vi "Service Key.vi"(11 "Service In":refnum<class "Service.lvclass">) -> (2 "Service Key":string, 3 "Service":refnum<class "Service.lvclass">)   [LabVIEW 2020, in "HTTP Server.lvlib" / "Values.lvclass"]
uses:
  Values.lvclass
  Service/Service.lvclass
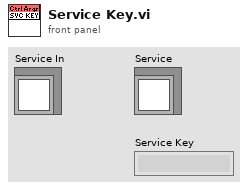
[diagram p1: front panel]
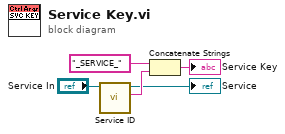
[diagram p0: block diagram]
diagram:
  n1 = call-dynamic "Service ID.vi"("Service in"="Service In") -> ("Service ID"=w4:string, "Service out"=→"Service":refnum<class "Service.lvclass">)  [unwired: 8 in, 1 out]
  n2 = Concatenate Strings("_SERVICE_" ("string"), w4) -> (→"Service Key":string)
